vi "Beam_Pointing_input.vi"() -> ()   [LabVIEW 2010]
panel:
  in  "Horizontal Beam pointing direction":dbl
  in  "Beams Pointing":T1(ring)
  out "Message":string
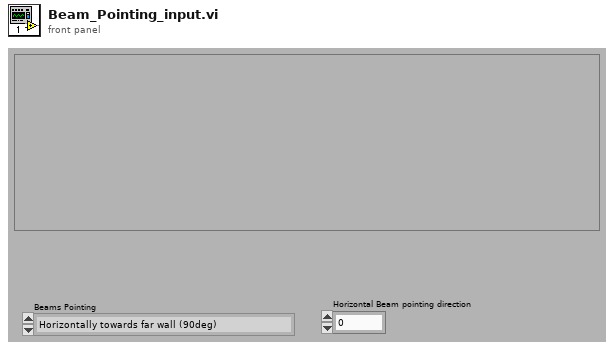
[diagram p1: front panel]
types:
  T1 = enum16{"Horizontally towards far wall (90deg)", "Horizontally upsteam (180deg)", "Horizontally towards windows (-90deg)", "Horizontal Please specify", "Vertical downwards"}
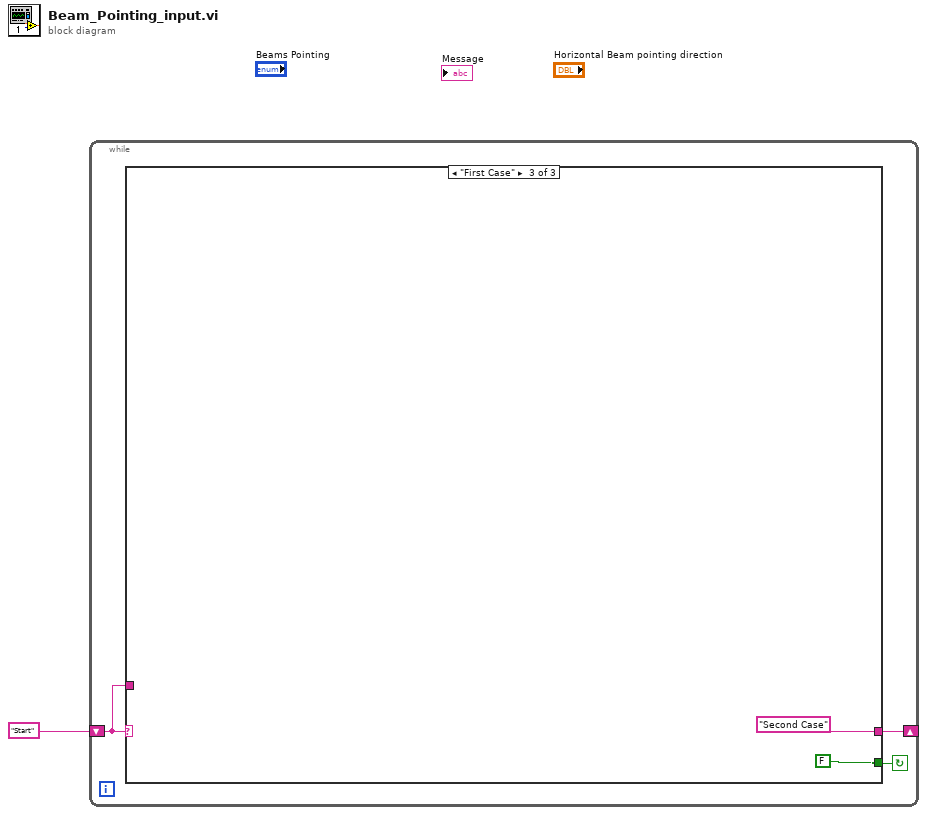
[diagram p0: block diagram]
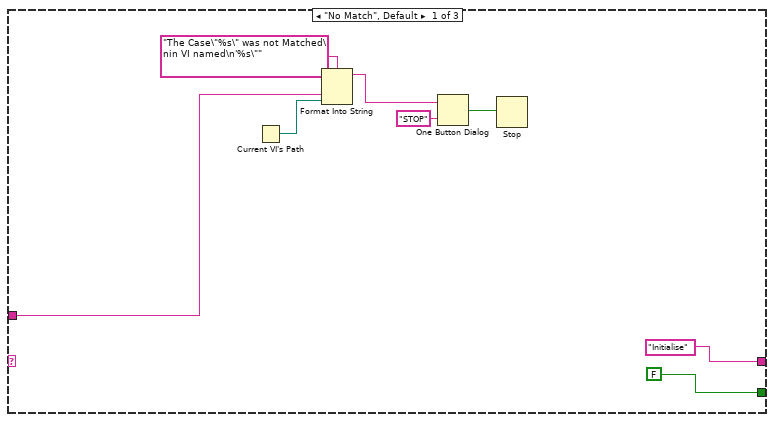
[diagram p2: hidden frame]
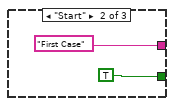
[diagram p3: hidden frame]
diagram:
  n1 = while {
    shift-left: "Start" -> [w2]
    shift-right: [w3] -> _
    stop <- w4 continue-if-true
    n2 = case shown="\"First Case\"" w2 {
      tunnel: [FALSE TRUE FALSE] -> w4
      tunnel: ["Initialise" "First Case" "Second Case"] -> w3
      tunnel: w2 -> [w7 _ _]
      frame "No Match", Default {
        n3 = Current VI's Path() -> (path=w6:path)
        n4 = Format Into String(format string="The Case\"%s\" was not Matched\nin VI named\n'%s\"" ("Format String"), w7, w6) -> (resulting string=w10:string)  [unwired: 2 in, 1 out]
        n5 = One Button Dialog(message=w10, button name ("OK")="STOP") -> (true=w8:bool)
        n6 = Stop(stop? (T)=w8) -> ()
      }
      frame "Start" {
      }
      frame "First Case" {
      }
    }
  }
